vi "obliczenia kursora.vi"(8 "error in (no error)":errorcluster, 11 "Wykres Ref":refnum<vi>) -> (0 "error out":errorcluster, 2 "Data":T1)   [LabVIEW 2013]
doc: "Oblicza różnicę między wartościami X i Y dwóch kursorów\ntypu single.\nNajpierw następuje sprawdzenie, czy istnieją dwa kursory typu single\na później zostaną wybrane dwa pierwsze z tabeli"
uses:
  Kontrolki/GUI/Wysw_kursorow.ctl
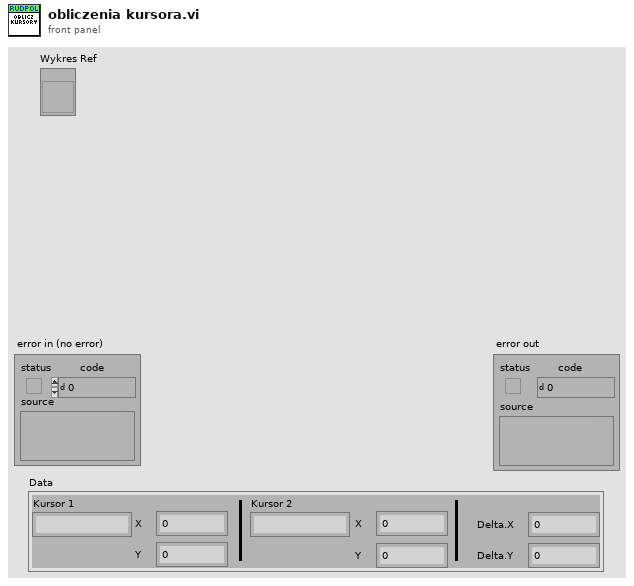
[diagram p1: front panel]
types:
  T1 = typedef "Wysw_kursorow.ctl" = cluster{"Pos.X1":dbl, "Pos.Y1":dbl, "Pos.X2":dbl, "Pos.Y2":dbl, "Delta.X":dbl, "Delta.Y":dbl, "Nazwa.1":string, "Nazwa.2":string}
  T2 = typedef "LVCursorListTypeDef.ctl" = cluster{"Name":string, "Color":u32, "Style":u8, "Point Style":u8, "Name Visible":bool, "Allow Drag":bool, "Cursor Mode":u32, "Plot":i32, "Index":i32, "Position":cluster{"X":dbl, "Y":dbl}, "X Scale":u32, "Y Scale":u32, "Watch Plots":i32[], "Watch All Plots":bool, "Plot Area":i32, "Label Offset":cluster{"X":dbl, "Y":dbl}}[]
  T3 = cluster{"Name":string, "Color":u32, "Style":u8, "Point Style":u8, "Name Visible":bool, "Allow Drag":bool, "Cursor Mode":u32, "Plot":i32, "Index":i32, "Position":cluster{"X":dbl, "Y":dbl}, "X Scale":u32, "Y Scale":u32, "Watch Plots":i32[], "Watch All Plots":bool, "Plot Area":i32, "Label Offset":cluster{"X":dbl, "Y":dbl}}
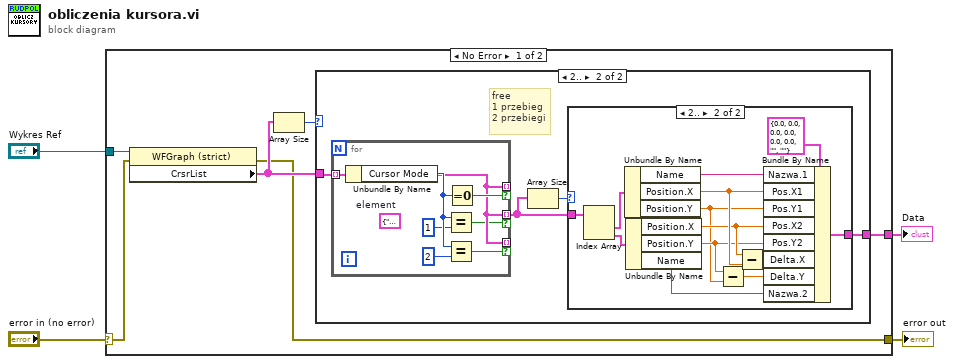
[diagram p0: block diagram]
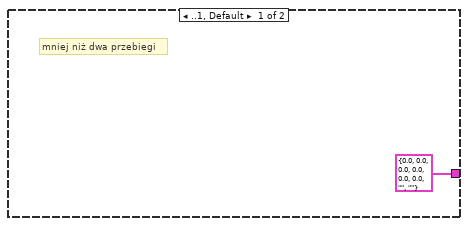
[diagram p2: hidden frame]
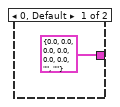
[diagram p3: hidden frame]
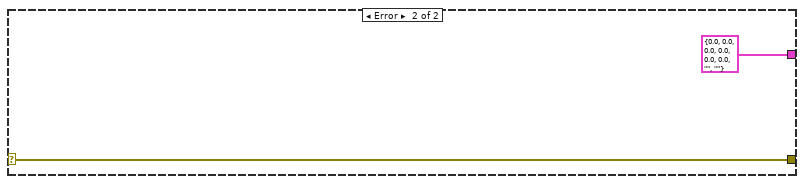
[diagram p4: hidden frame]
diagram:
  n1 = case shown="No Error" "error in (no error)" {
    selector: "error in (no error)" -> [w9 w38]
    tunnel: [w6 w38] -> w3
    tunnel: "Wykres Ref" -> [w10 _]
    tunnel: [w5 T1 {"Pos.X1"=0.0, "Pos.Y1"=0.0, "Pos.X2"=0.0, "Pos.Y2"=0.0, "Delta.X"=0.0, "Delta.Y"=0.0, "Nazwa.1"="", "Nazwa.2"=""}] -> w1
    frame No Error {
      n2 = property class="WFGraph (strict)"(reference=w10, error in=w9) -> (error out=w6:errorcluster, "CrsrList"=w7:T2)  [unwired: 1 out]
      n3 = Array Size(array=w7) -> (size(s)=w8:i32)
      n4 = case shown="2.." w8 {
        tunnel: w7 -> [_ w15]
        tunnel: [T1 {"Pos.X1"=0.0, "Pos.Y1"=0.0, "Pos.X2"=0.0, "Pos.Y2"=0.0, "Delta.X"=0.0, "Delta.Y"=0.0, "Nazwa.1"="", "Nazwa.2"=""} w12] -> w5
        frame ..1, Default {
          # "mniej niż dwa przebiegi"
        }
        frame 2.. {
          # "free\n1 przebieg\n2 przebiegi"
          n5 = for {
            tunnel: w15 -> [w32] mode=indexing
            tunnel: [w32] -> _ mode=indexing if=w33
            tunnel: [w32] -> w13 mode=indexing if=w31
            tunnel: [w32] -> _ mode=indexing if=w30
            (unwired) T3 {"Name"="", "Color"=0, "Style"=0, "Point Style"=0, "Name Visible"=FALSE, "Allow Drag"=FALSE, "Cursor Mode"=0, "Plot"=0, "Index"=0, "Position"={"X"=0.0, "Y"=0.0}, "X Scale"=0, "Y Scale"=0, "Watch Plots"=[], "Watch All Plots"=FALSE, "Plot Area"=0, "Label Offset"={"X"=0.0, "Y"=0.0}}  # element
            n6 = Unbundle By Name(w32) -> ("Cursor Mode"=w36:u32)
            n7 = Equal?(x=w36, y=u32 1) -> (x = y?=w31:bool)
            n8 = Equal?(x=w36, y=u32 2) -> (x = y?=w30:bool)
            n9 = Equal To 0?(x=w36) -> (x = 0?=w33:bool)
          }
          n10 = Array Size(array=w13) -> (size(s)=w14:i32)
          n11 = case shown="2.." w14 {
            tunnel: w13 -> [_ w29]
            tunnel: [T1 {"Pos.X1"=0.0, "Pos.Y1"=0.0, "Pos.X2"=0.0, "Pos.Y2"=0.0, "Delta.X"=0.0, "Delta.Y"=0.0, "Nazwa.1"="", "Nazwa.2"=""} w24] -> w12
            frame 0, Default {
            }
            frame 2.. {
              n12 = Index Array(array=w29) -> (element #1=w28:T3, element #2=w27:T3)  [unwired: 2 in]
              n13 = Unbundle By Name(w28) -> ("Name"=w17:string, "Position.X"=w23:dbl, "Position.Y"=w20:dbl)
              n14 = Unbundle By Name(w27) -> ("Position.X"=w22:dbl, "Position.Y"=w21:dbl, "Name"=w18:string)
              n15 = Subtract(x=w21, y=w20) -> (x-y=w25:dbl)
              n16 = Subtract(x=w22, y=w23) -> (x-y=w26:dbl)
              n17 = Bundle By Name(cluster=T1 {"Pos.X1"=0.0, "Pos.Y1"=0.0, "Pos.X2"=0.0, "Pos.Y2"=0.0, "Delta.X"=0.0, "Delta.Y"=0.0, "Nazwa.1"="", "Nazwa.2"=""}, "Nazwa.1"=w17, "Pos.X1"=w23, "Pos.Y1"=w20, "Pos.X2"=w22, "Pos.Y2"=w21, "Delta.X"=w26, "Delta.Y"=w25, "Nazwa.2"=w18) -> (w24:T1)
            }
          }
        }
      }
    }
    frame Error {
    }
  }
  "error out" <- w3
  "Data" <- w1
